vi "Save Block Diagram.vi"(8 "error in (no error)":errorcluster, 10 "path":path, 11 "vi ref":refnum<vi>) -> (0 "error out":errorcluster, 1 "unavailable":bool, 2 "path out":path, 3 "reference out":refnum<vi>)   [LabVIEW 2014, in "lvprj2html.lvlib"]
uses:
  lvprj2html.lvlib
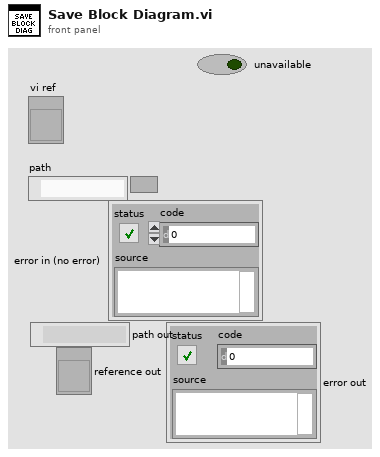
[diagram p1: front panel]
types:
  T1 = enum32{"invalid VI type", "Standard VI", "Control VI", "Global VI", "Polymorphic VI", "Configuration VI", "SubSystem", "Facade VI", "Method VI", "Statechart Diagram VI"}
  T2 = typedef "imagedata.ctl" = cluster{"image type":i32, "image depth":i32, "image":u8[], "mask":u8[], "colors":u32[], "Rectangle":cluster{"left":i16, "top":i16, "right":i16, "bottom":i16}}
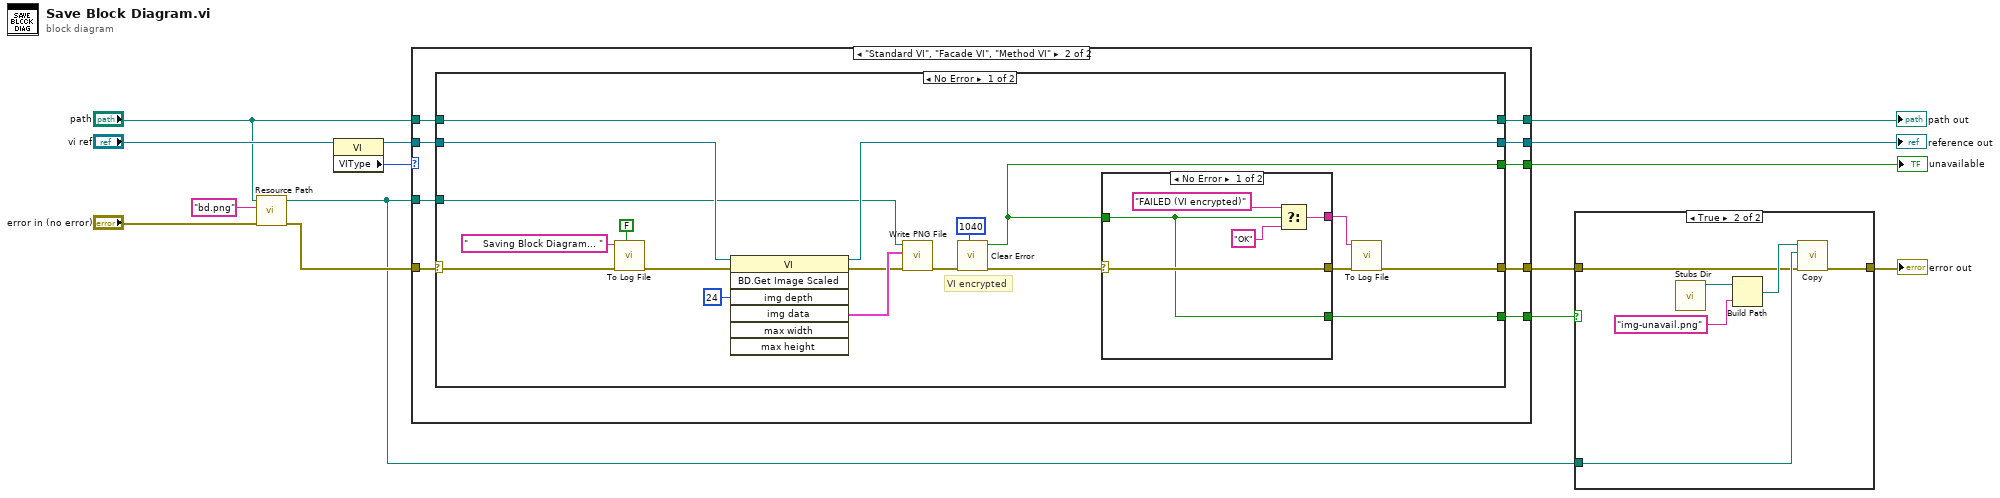
[diagram p0: block diagram]
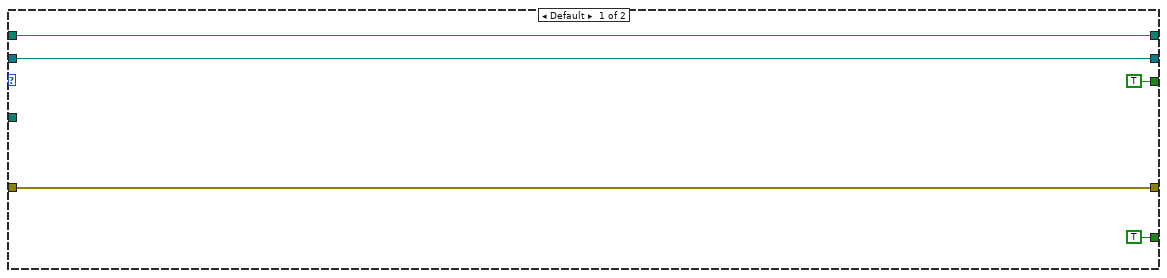
[diagram p3: hidden frame]
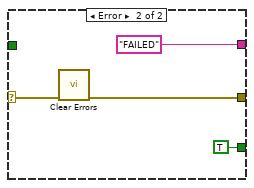
[diagram p4: hidden frame]
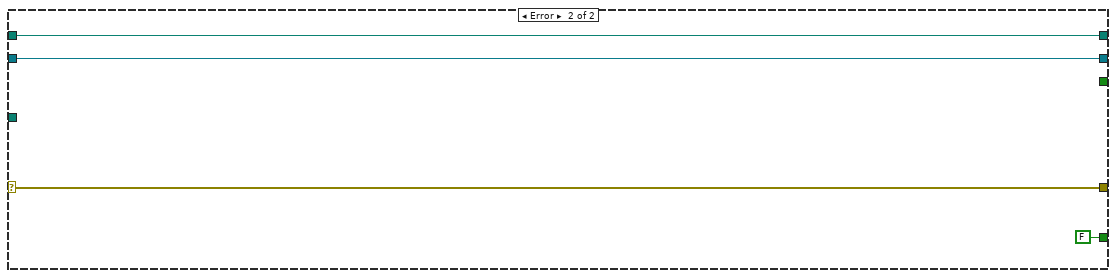
[diagram p5: hidden frame]
diagram:
  n1 = call "Resource Path.vi"("error in (no error)"="error in (no error)", "resource file name"="bd.png", "data dir"="path") -> ("error out"=w5:errorcluster, "path"=w3:path)  [unwired: 7 in]
  n2 = property class="VI"(reference="vi ref") -> (reference out=w10:refnum<vi>, "VIType"=w9:T1)  [unwired: 1 in, 1 out]
  n3 = case shown="\"Standard VI\", \"Facade VI\", \"Method VI\"" w9 {
    tunnel: "path" -> [w19 w28]
    tunnel: [w18 w27] -> w14
    tunnel: [w16 w26] -> w2
    tunnel: [TRUE ("clear") w25] -> w13
    tunnel: w5 -> [w16 w24]
    tunnel: [w19 w23] -> w12
    tunnel: w10 -> [w18 w22]
    tunnel: w3 -> [_ w21]
    tunnel: [TRUE ("clear") w20] -> w4
    frame Default {
    }
    frame "Standard VI", "Facade VI", "Method VI" {
      n4 = case shown="No Error" w24 {
        selector: w24 -> [w37 w60]
        tunnel: w22 -> [w47 w59]
        tunnel: w28 -> [w36 w58]
        tunnel: [w42 w59] -> w27
        tunnel: [w32 w60] -> w26
        tunnel: [w38 _] -> w25
        tunnel: [w36 w58] -> w23
        tunnel: w21 -> [w30 _]
        tunnel: [w29 FALSE ("clear")] -> w20
        frame No Error {
          # "VI encrypted"
          n5 = call "To Log File.vi"("new line"=FALSE, "error in (no error)"=w37, "string"="     Saving Block Diagram... " ("format string")) -> ("error out"=w40:errorcluster)  [unwired: 8 in]
          n6 = invoke class="VI" method="BD.Get Image Scaled"(reference=w47, error in=w40, "img depth"=24 ("Image Depth")) -> (reference out=w42:refnum<vi>, error out=w31:errorcluster, "img data"=w44:T2)  [unwired: 4 in, 4 out]
          n7 = call <vilib>:"Write PNG File.vi"("error in (no error)"=w31, "image data"=w44, "path to PNG file"=w30) -> ("error out"=w45:errorcluster)  [unwired: 7 in, 1 out]
          n8 = call "Clear Error.vi"("code"=1040, "error in (no error)"=w45) -> ("error out"=w35:errorcluster, "clear"=w38:bool)  [unwired: 8 in]
          n9 = case shown="No Error" w35 {
            selector: w35 -> [w50 w56]
            tunnel: [w50 w54] -> w33
            tunnel: w38 -> [w48 _]
            tunnel: [w49 "FAILED" ("string")] -> w34
            tunnel: [w48 TRUE ("clear")] -> w29
            frame No Error {
              n10 = Select(t="FAILED (VI encrypted)" ("format string"), s=w48, f="OK" ("format string")) -> (s? t:f=w49:string)
            }
            frame Error {
              n11 = call <vilib>:"Clear Errors.vi"("error in (no error)"=w56) -> ("error out"=w54:errorcluster)  [unwired: 5 in, 1 out]
            }
          }
          n12 = call "To Log File.vi"("error in (no error)"=w33, "string"=w34) -> ("error out"=w32:errorcluster)  [unwired: 9 in]
        }
        frame Error {
        }
      }
    }
  }
  "unavailable" <- w13
  "path out" <- w12
  "reference out" <- w14
  n13 = case shown="True" w4 {
    tunnel: w3 -> [_ w64]
    tunnel: w2 -> [w61 w63]
    tunnel: [w61 w62] -> w1
    frame False {
    }
    frame True {
      n14 = call "Stubs Dir.vi"() -> ("path"=w65:path)  [unwired: 11 in]
      n15 = Build Path(base path=w65, name or relative path="img-unavail.png") -> (appended path=w67:path)
      n16 = call "Copy.vi"("error in (no error)"=w63, "dst"=w64, "src"=w67) -> ("error out"=w62:errorcluster)  [unwired: 8 in]
    }
  }
  "error out" <- w1
